vi "Set MB Registers.vi"(8 "error in (no error)":errorcluster, 9 "Register Data":dbl[](array[numeric]), 10 "Register Names":string[](array[string]), 11 "HPS17K IP Address":string) -> (0 "error out":errorcluster, 3 "Register Data":string[][](array[string]))   [LabVIEW 2023, in "HPS-17000-PowerModule.lvlib" / "HPS-17000-PowerModule.lvclass"]
uses:
  <vilib>/net/SSH/Client/PuTTY/PuTTY Client.lvclass
  <vilib>/net/SSH/Client/Generic/Generic Client.lvclass/Generic Client.ctl
  <vilib>/net/SSH/Client/Generic/Write trust on first use.vi
  <vilib>/Utility/error.llb/Trim Whitespace One-Sided.vi
  HPS-17000-PowerModule.lvclass
  HPS-17000-PowerModule.lvclass/HPS-17000-PowerModule.ctl
  <vilib>/net/SSH/NI_SSH.lvlib
  C:/Program Files/National Instruments/LabVIEW 2023/vi.lib/net/SSH/Client/Generic/Generic Client.lvclass
  C:/Program Files/National Instruments/LabVIEW 2023/vi.lib/net/SSH/Client/PuTTY/PuTTY Client.lvclass
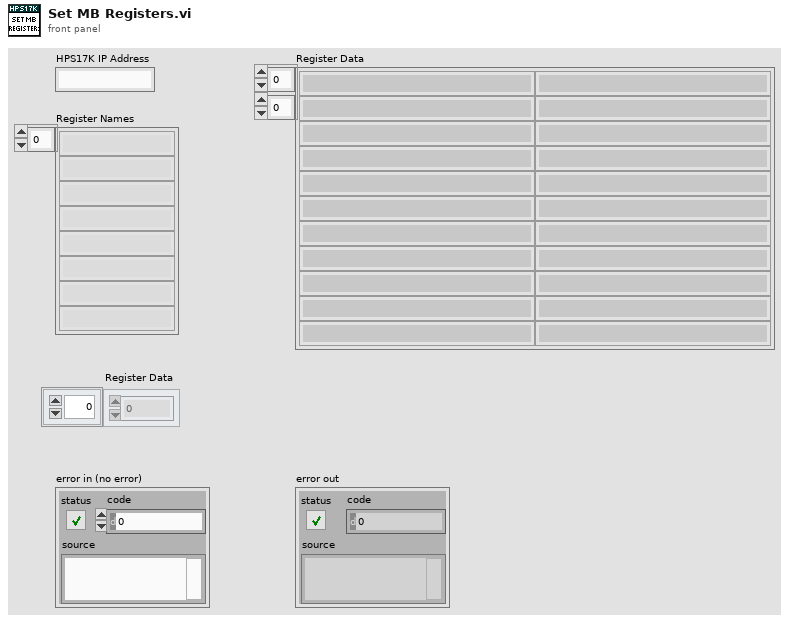
[diagram p1: front panel]
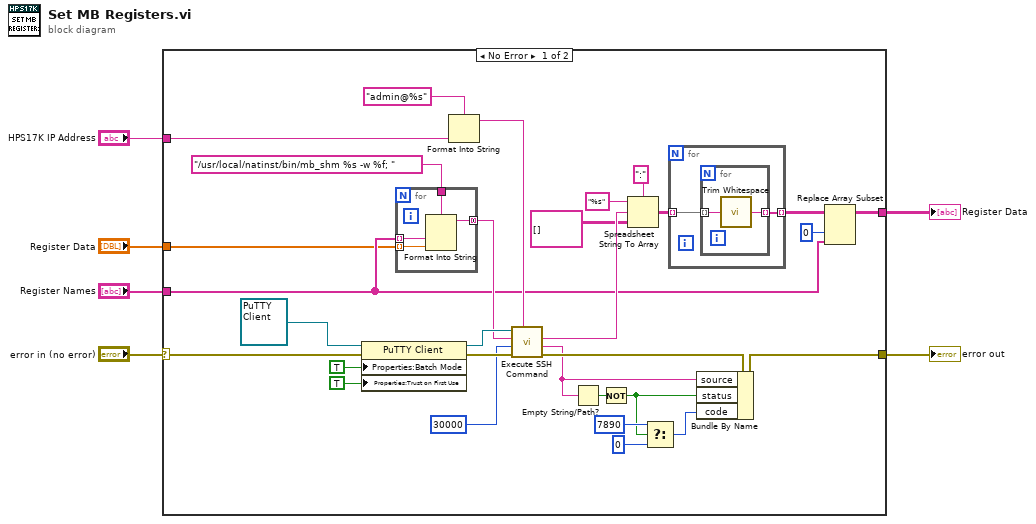
[diagram p0: block diagram]
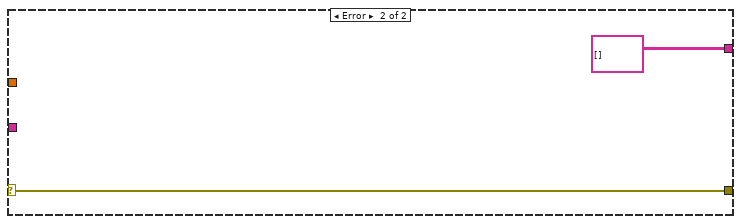
[diagram p2: hidden frame]
diagram:
  n1 = case shown="No Error" "error in (no error)" {
    selector: "error in (no error)" -> [w35 w46]
    tunnel: "HPS17K IP Address" -> [w36 _]
    tunnel: [w10 string[][] []] -> w5
    tunnel: [w17 w46] -> w4
    tunnel: "Register Names" -> [w8 _]
    tunnel: "Register Data" -> [w7 _]
    frame No Error {
      n2 = property class="PuTTY Client"(reference=refnum<class "PuTTY Client.lvclass"> refnum ("NI_SSH.lvlib:PuTTY Client"), error in=w35, "Properties:Batch Mode"=TRUE ("Batch Mode"), "Properties:Trust on First Use"=TRUE ("Trust on First Use")) -> (reference out=w33:refnum<class "PuTTY Client.lvclass">, error out=w32:errorcluster)
      n3 = for {
        tunnel: w8 -> [w44] mode=indexing
        tunnel: "/usr/local/natinst/bin/mb_shm %s -w %f; " ("format string") -> [w43]
        tunnel: [w42] -> w25 mode=concatenating
        tunnel: w7 -> [w41] mode=indexing
        n4 = Format Into String(format string=w43, w44, w41) -> (resulting string=w42:string)  [unwired: 2 in, 1 out]
      }
      n5 = Format Into String(format string="admin@%s", w36) -> (resulting string=w34:string)  [unwired: 2 in, 1 out]
      n6 = call <vilib>:"Execute SSH Command.vi"("user@host"=w34, "error in (no error)"=w32, "timeout (ms)"=30000, "command line"=w25, "session in"=w33) -> ("error out"=w20:errorcluster, "standard error"=w18:string, "standard output"=w22:string)  [unwired: 2 in, 2 out]
      n7 = Empty String/Path?(string/path=w18) -> (empty?=w19:bool)
      n8 = Not(x=w19) -> (.not. x?=w15:bool)
      n9 = Spreadsheet String To Array(delimiter (Tab)=":", format string="%s", spreadsheet string=w22, array type (2D Dbl)=string[][] []) -> (array=w12:string[][])
      n10 = Select(t=7890 ("code"), s=w15, f=0) -> (s? t:f=w14:i32)
      n11 = for {
        tunnel: w12 -> [w38] mode=indexing
        tunnel: [w37] -> w11 mode=indexing
        n12 = for {
          tunnel: w38 -> [w40] mode=indexing
          tunnel: [w39] -> w37 mode=indexing
          n13 = call <vilib>:"Trim Whitespace.vi"("string"=w40) -> ("trimmed string"=w39:string)  [unwired: 1 in]
        }
      }
      n14 = Bundle By Name(cluster=w20, "source"=w18, "status"=w15, "code"=w14) -> (w17:errorcluster)
      n15 = Replace Array Subset(array=w11, new element=w8, index (col)=0 ("disabled index (col)")) -> (w10:string[][])  [unwired: 1 in]
    }
    frame Error {
    }
  }
  "Register Data" <- w5
  "error out" <- w4
